vi "MouseButtonUp.vi"(4 "Position":T1, 6 "Button":u8, 7 "Clicks":u8, 8 "error in (no error)":errorcluster, 9 "Which":T2, 10 "Timestamp":u64, 11 "WindowEventInterface in":refnum<class "WindowEventInterface.lvclass">) -> (0 "error out":errorcluster)   [LabVIEW 2020, in "GLF.lvlib" / "WindowEventInterface.lvclass"]
uses:
  WindowEventInterface.lvclass
  <vilib>/Saukko/LV SDL3/Sources/SDL3/Mouse/MouseID--integer.ctl
  <vilib>/Saukko/LV SDL3/Sources/SDL3/Mouse/Mouse.lvlib
  <vilib>/Saukko/LV SDL3/Sources/SDL3/Rect/FPoint--cluster.ctl
  <vilib>/Saukko/LV SDL3/Sources/SDL3/Rect/Rect.lvlib
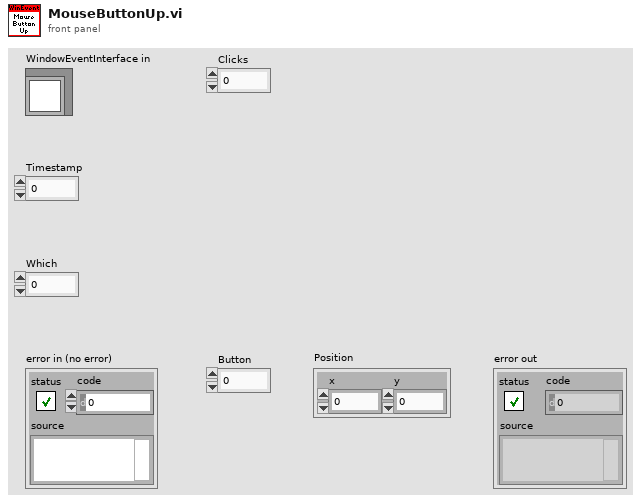
[diagram p1: front panel]
types:
  T1 = typedef "SDL3.lvlib/Rect.lvlib/FPoint--cluster.ctl" = cluster{"x":sgl, "y":sgl}
  T2 = typedef "SDL3.lvlib/Mouse.lvlib/MouseID--integer.ctl" = u32
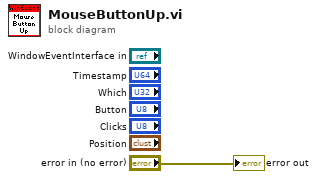
[diagram p0: block diagram]
diagram:
  "error out" <- "error in (no error)"
